vi "Flatten Label Values.vi"(5 "Label Values":string[](array[string])) -> (2 "Flattened labelvalues":string)   [LabVIEW 2020, in "Metrics.lvlib" / "Metric.lvclass"]
uses:
  Metric.lvclass
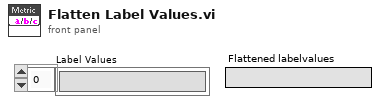
[diagram p1: front panel]
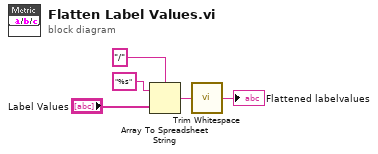
[diagram p0: block diagram]
diagram:
  n1 = Array To Spreadsheet String(delimiter (Tab)="/", array="Label Values", 3:"%s" ("format string")) -> (spreadsheet string=w3:string)
  n2 = call <vilib>:"Trim Whitespace.vi"("string"=w3) -> ("trimmed string"=→"Flattened labelvalues":string)  [unwired: 1 in]
